vi "StartandConnectCore.vi"(8 "error in (no error)":errorcluster, 10 "Service Details":T1, 11 "MicronClient in":refnum<class "MicronClient.lvclass">) -> (0 "error out":errorcluster, 3 "MicronClient out":refnum<class "MicronClient.lvclass">)   [LabVIEW 2019, in "MicronClient.lvclass"]
uses:
  MicronClient.lvclass
  Typedefs/Service Details.ctl
  b3105294-9a6f-41a1-b30d-198c4dc4b55b.vi
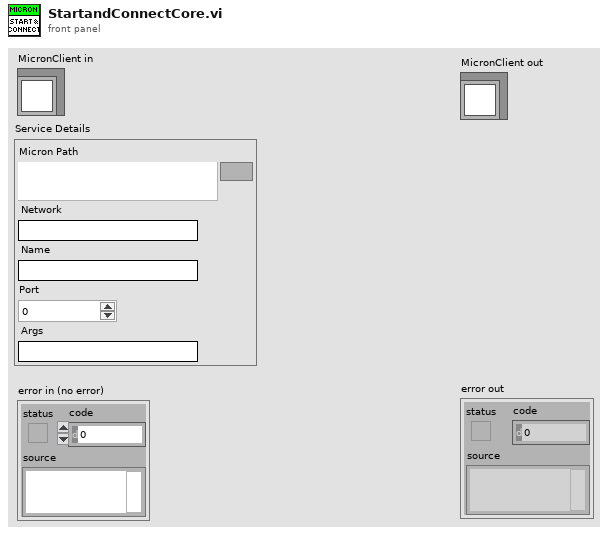
[diagram p1: front panel]
types:
  T1 = typedef "MicronClient.lvclass/Service Details.ctl" = cluster{"Micron Path":path, "Network":string, "Name":string, "Port":i32, "Args":string}
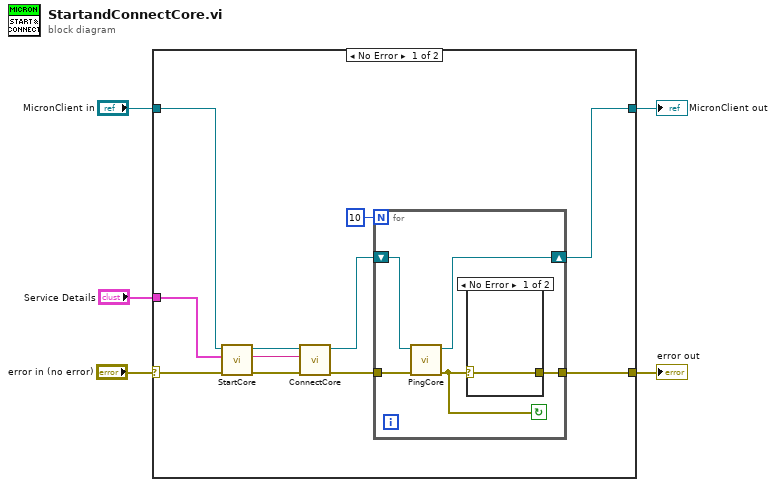
[diagram p0: block diagram]
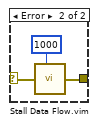
[diagram p2: hidden frame]
diagram:
  n1 = case shown="No Error" "error in (no error)" {
    selector: "error in (no error)" -> [w10 w27]
    tunnel: [w8 w27] -> w4
    tunnel: [w9 w26] -> w2
    tunnel: "MicronClient in" -> [w12 w26]
    tunnel: "Service Details" -> [w11 _]
    frame No Error {
      n2 = call-dynamic "StartCore.vi"("error in (no error)"=w10, "Service Details"=w11, "MicronClient in"=w12) -> ("error out"=w16:errorcluster, "Connection String"=w7:string, "MicronClient out"=w14:refnum<class "MicronClient.lvclass">)  [unwired: 6 in]
      n3 = call-dynamic "ConnectCore.vi"("error in (no error)"=w16, "Connection String"=w7, "MicronClient in"=w14) -> ("error out"=w15:errorcluster, "MicronClient out"=w13:refnum<class "MicronClient.lvclass">)  [unwired: 7 in]
      n4 = for {
        N: 10 -> [_]
        shift-right: [w19] -> w9
        shift-left: w13 -> [w20]
        tunnel: w15 -> [w21]
        tunnel: [w17] -> w8
        stop <- w18 continue-if-true
        n5 = call-dynamic "PingCore.vi"("error in (no error)"=w21, "MicronClient in"=w20) -> ("error out"=w18:errorcluster, "MicronClient out"=w19:refnum<class "MicronClient.lvclass">)  [unwired: 7 in, 1 out]
        n6 = case shown="No Error" w18 {
          selector: w18 -> [w22 w25]
          tunnel: [w22 w24] -> w17
          frame No Error {
          }
          frame Error {
            n7 = call "Stall Data Flow.vim"("value in"=w25, "milliseconds to wait"=u32 1000) -> ("value out"=w24:errorcluster)  [unwired: 1 out]
          }
        }
      }
    }
    frame Error {
    }
  }
  "error out" <- w4
  "MicronClient out" <- w2
